vi "Lines Filter-#.vi"(8 "error in (no error)":errorcluster, 11 "Lines":string[](array[string])) -> (0 "error out":errorcluster, 3 "Config Text List":string[](array[string]))   [LabVIEW 2020]
doc: "[Covers: REQ-KeyPoint-I-CommentInBarcodeFile]\n[Covers: REQ-KeyPoint-I-CommentInEnv_Config]\n[Covers: REQ-KeyPoint-I-CommentInRecipe]"
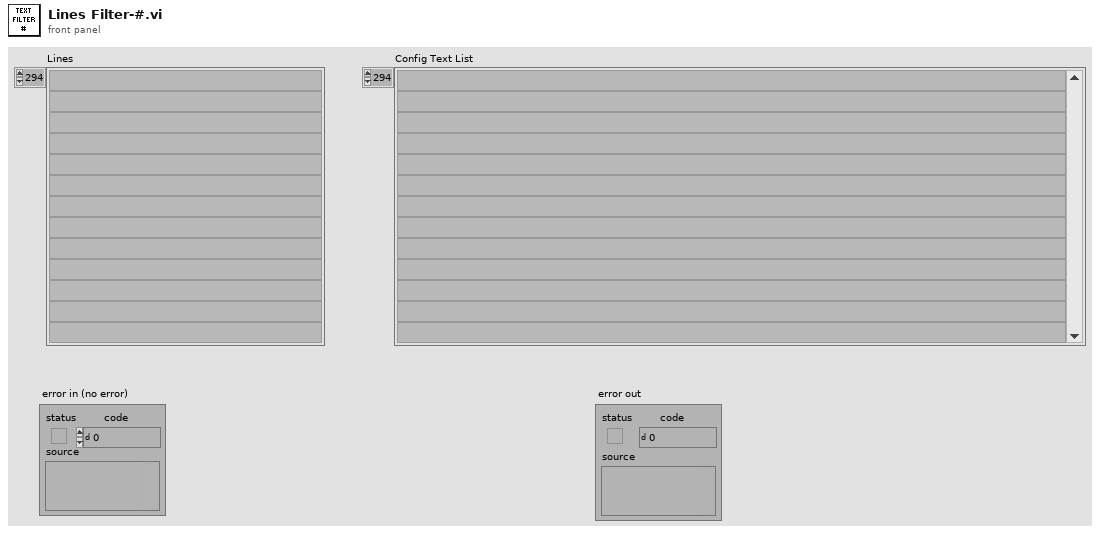
[diagram p1: front panel]
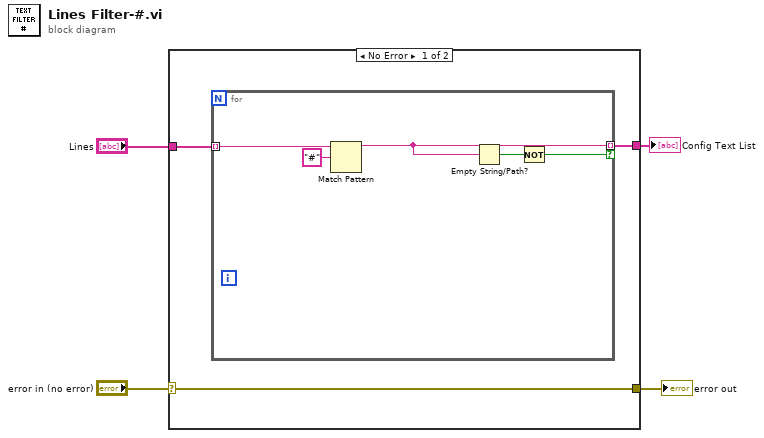
[diagram p0: block diagram]
diagram:
  n1 = case shown="No Error" "error in (no error)" {
    selector: "error in (no error)" -> [w5 w13]
    tunnel: [w5 w13] -> w3
    tunnel: "Lines" -> [w7 _]
    tunnel: [w6 _] -> w1
    frame No Error {
      n2 = for {
        tunnel: w7 -> [w10] mode=indexing
        tunnel: [w8] -> w6 mode=indexing if=w11
        n3 = Match Pattern(string=w10, regular expression="#") -> (before substring=w8:string)  [unwired: 1 in, 3 out]
        n4 = Empty String/Path?(string/path=w8) -> (empty?=w9:bool)
        n5 = Not(x=w9) -> (.not. x?=w11:bool)
      }
    }
    frame Error {
    }
  }
  "error out" <- w3
  "Config Text List" <- w1
